vi "Append Ordered Array.vi"(8 "error in (no error)":errorcluster, 10 "Ordered Array 2 in":refnum<class "Ordered Array.lvclass">, 11 "Ordered Array in":refnum<class "Ordered Array.lvclass">) -> (0 "error out":errorcluster, 3 "Ordered Array out":refnum<class "Ordered Array.lvclass">)   [LabVIEW 2019, in "Ordered Array.lvclass"]
uses:
  Ordered Array.lvclass
  Ordered Array.lvclass/Ordered Array.ctl
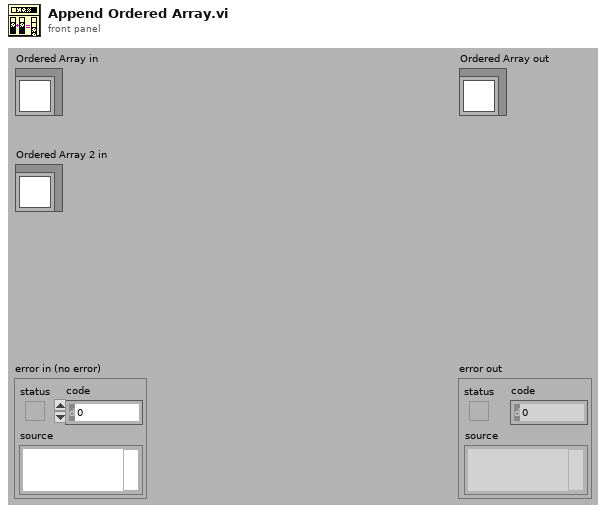
[diagram p1: front panel]
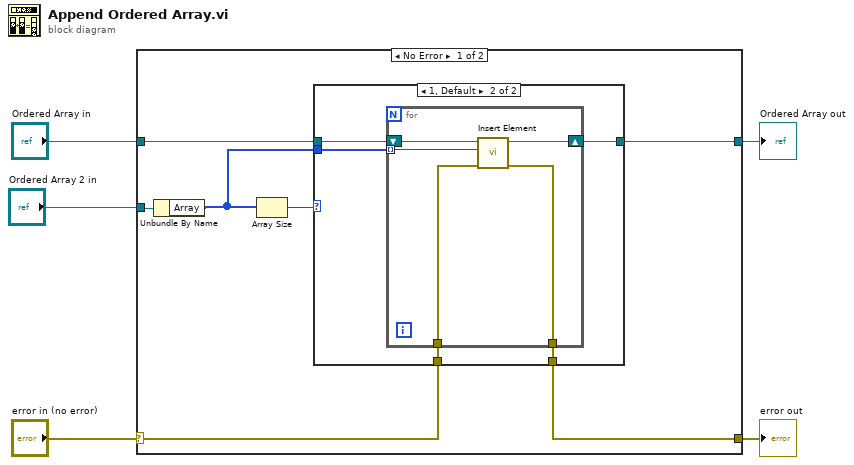
[diagram p0: block diagram]
diagram:
  n1 = case shown="No Error" "error in (no error)" {
    selector: "error in (no error)" -> [w7 w26]
    tunnel: [w6 w26] -> w4
    tunnel: [w11 w25] -> w1
    tunnel: "Ordered Array in" -> [w12 w25]
    tunnel: "Ordered Array 2 in" -> [w9 _]
    frame No Error {
      n2 = Unbundle By Name(w9) -> ("Array"=w8:u32[])
      n3 = Array Size(array=w8) -> (size(s)=w10:i32)
      n4 = case shown="1, Default" w10 {
        tunnel: [w13 w17] -> w11
        tunnel: w8 -> [_ w19]
        tunnel: w12 -> [w13 w18]
        tunnel: w7 -> [w14 w16]
        tunnel: [w14 w15] -> w6
        frame 0 {
        }
        frame 1, Default {
          n5 = for {
            tunnel: w19 -> [w23] mode=indexing
            tunnel: w16 -> [w21]
            tunnel: [w20] -> w15
            shift-right: [w22] -> w17
            shift-left: w18 -> [w24]
            n6 = call "Insert Element.vi"("error in (no error)"=w21, "Element"=w23, "Ordered Array in"=w24) -> ("error out"=w20:errorcluster, "Ordered Array out"=w22:refnum<class "Ordered Array.lvclass">)  [unwired: 7 in]
          }
        }
      }
    }
    frame Error {
    }
  }
  "error out" <- w4
  "Ordered Array out" <- w1
